vi "PIDTuner.vi"() -> ()   [LabVIEW 2017]
uses:
  <vilib>/addons/control/pid/pid.llb/PID (DBL).vi
  <vilib>/addons/control/pid/NI_PID_pid.lvlib
panel:
  in  "setpoint":dbl format="%.2f"
  in  "PID gains":T1={"proportional gain (Kc)"=1.0, "integral time (Ti, min)"=0.01, "derivative time (Td, min)"=0.0} {"derivative time (Td, min)" format="%.7f"; "integral time (Ti, min)" format="%.7f"; "proportional gain (Kc)" format="%.7f"}
  in  "stop":bool
  out "pot out":dbl(graph)
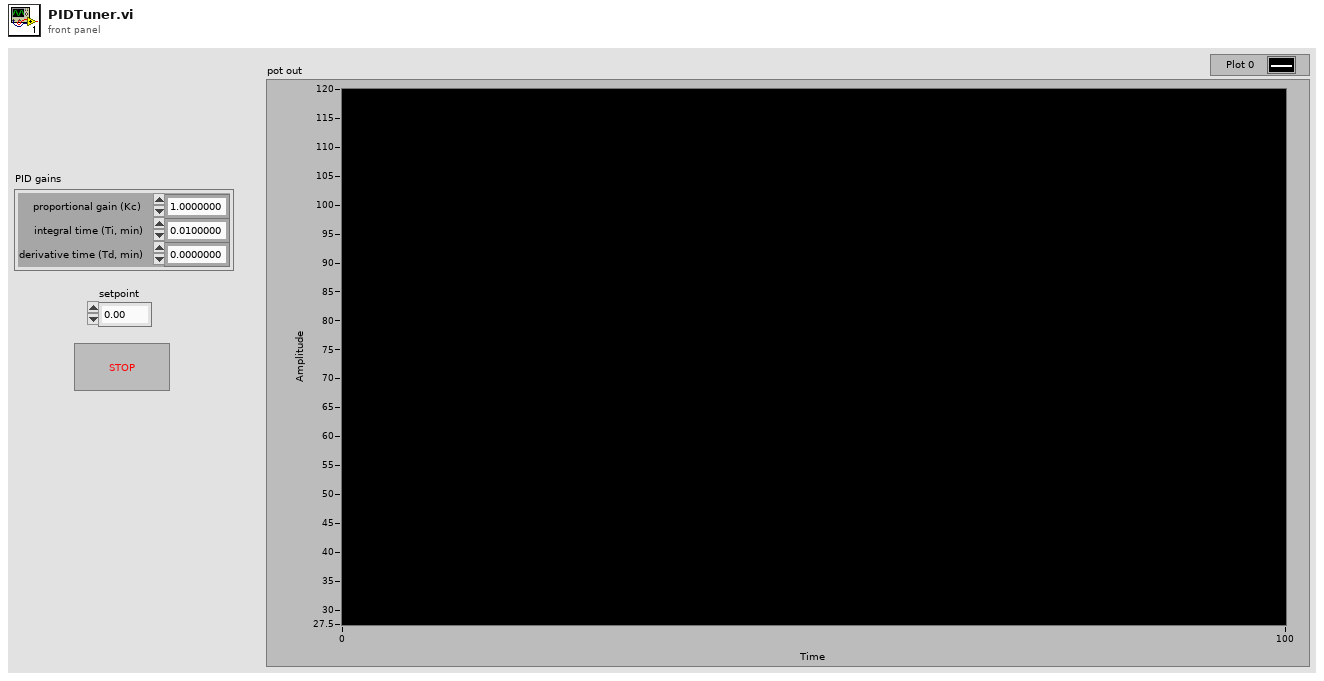
[diagram p1: front panel]
types:
  T1 = cluster{"proportional gain (Kc)":dbl, "integral time (Ti, min)":dbl, "derivative time (Td, min)":dbl}
  T2 = cluster{"static gain":dbl, "lag (s)":dbl, "deadtime (s)":dbl, "load":dbl, "deadband":dbl, "sensor noise":dbl, "initial PV":dbl, "plant noise":dbl}
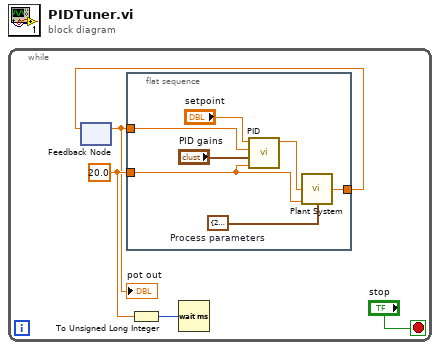
[diagram p0: block diagram]
diagram:
  n1 = while {
    stop <- "stop" stop-if-true
    w5 = 20.0 ("Sampling Time dt (s)")
    n2 = feedback-in #1(w2) -> ()
    n3 = feedback #1() -> (w1:dbl)  [unwired: 1 in]
    "pot out" <- w1
    n4 = flat-sequence {
      tunnel: [w12] -> w2
      tunnel: w5 -> [w8]
      tunnel: w1 -> [w6]
      frame #0 {
        w11 = T2 {"static gain"=2.5, "lag (s)"=100.0, "deadtime (s)"=0.01, "load"=0.0, "deadband"=0.0, "sensor noise"=0.0, "initial PV"=30.0, "plant noise"=0.0}  # Process parameters
        n5 = call-poly <vilib>:"PID.vi"("dt (s)"=w8, "PID gains"="PID gains", "process variable"=w6, "setpoint"="setpoint") -> ("output"=w10:dbl)  [unwired: 6 in, 1 out]
        n6 = call "Plant System.vi"("Plant Input"=w10, "dt (s)"=w8, "process parameters"=w11) -> ("Plant Output"=w12:dbl)  [unwired: 12 in]
      }
    }
    n7 = To Unsigned Long Integer(number=w5) -> (unsigned 32bit integer=w4:u32)
    n8 = Wait (ms)(milliseconds to wait=w4) -> ()  [unwired: 1 out]
  }
